vi "Properties Section Page.vi"(8 "error in (no error)":errorcluster, 11 "Node Ptr":T1 format="%.0x") -> (0 "error out":errorcluster)   [LabVIEW 2019, in "SLSC EDS System Explorer.lvlib"]
uses:
  SLSC EDS System Explorer.lvlib
  <vilib>/NI VeriStand/Custom Device API/Custom Device Item Ref.ctl
  Shared/Constants.vi
  <vilib>/NI VeriStand/Custom Device API/Custom Device API.lvlib
  Shared/SLSC EDS Shared.lvlib
panel:
  in  "SHDocVw.IWebBrowser":refnum<k7>(container)
  in  "Header 2":cluster{"Section Name":string}={"Section Name"="Properties Settings"}
  # "Name"
  # "Description"
  # "Datatype"
  # "Value"
  # "Min"
  # "Max"
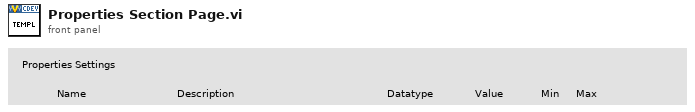
[diagram p1: front panel]
types:
  T1 = typedef "Custom Device API.lvlib/Custom Device Item Ref.ctl" = u64
  T2 = typedef "Custom Device API.lvlib/Custom Device Commands.ctl" = enum16{"Default", "Item renamed", "Shutdown", "Dynamic button pressed"}
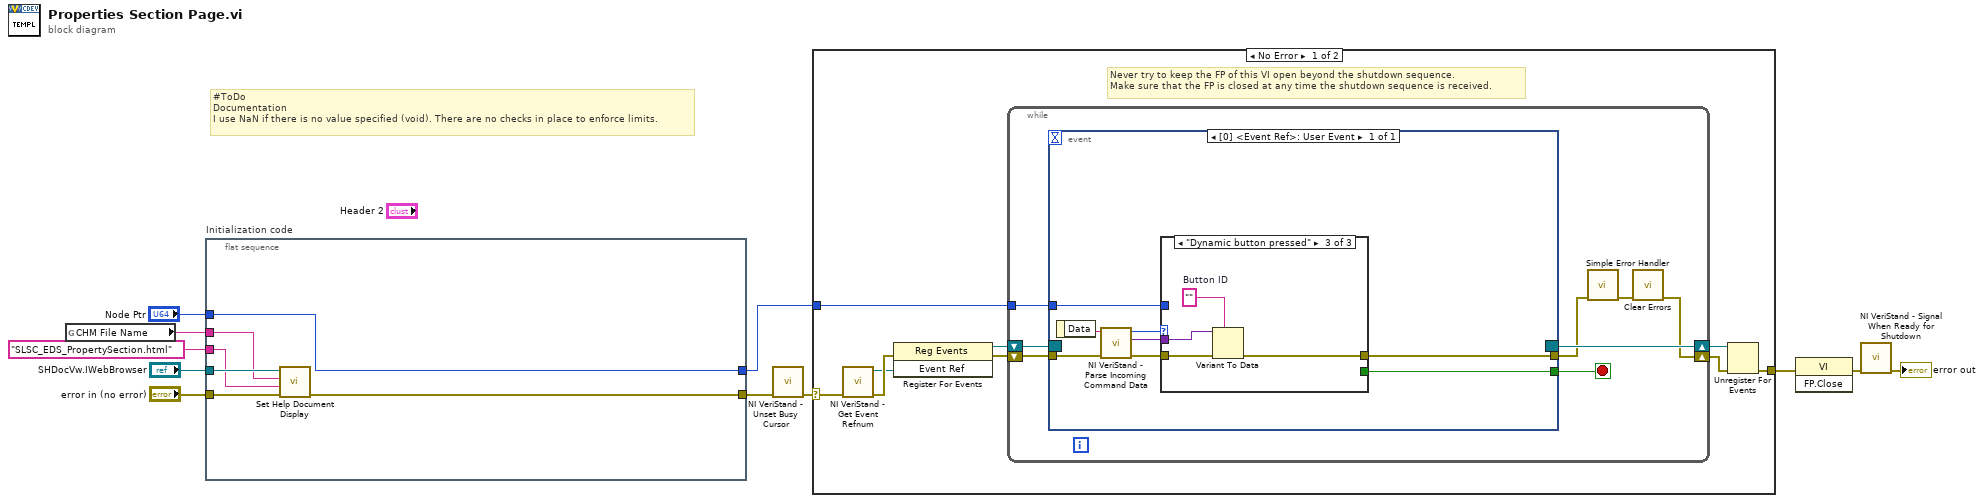
[diagram p0: block diagram]
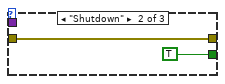
[diagram p3: hidden frame]
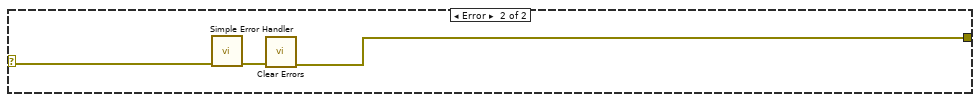
[diagram p4: hidden frame]
diagram:
  # "#ToDo\nDocumentation\nI use NaN if there is no value specified (void). There are no checks in place to enforce limits."
  n1 = global read "Constants.vi" "CHM File Name"() -> (w1:string)
  n2 = flat-sequence "Initialization code" {
    tunnel: "error in (no error)" -> [w17]
    tunnel: "Node Ptr" -> [w13]
    tunnel: [w12] -> w7
    tunnel: [w13] -> w4
    tunnel: "SHDocVw.IWebBrowser" -> [w16]
    tunnel: "SLSC_EDS_PropertySection.html" ("HTML File") -> [w15]
    tunnel: w1 -> [w14]
    frame #0 {
      n3 = call "Set Help Document Display.vi"("error in (no error)"=w17, "HTML File"=w15, "Main CHM File"=w14, "SHDocVw.IWebBrowser2"=w16) -> ("error out"=w12:errorcluster)  [unwired: 7 in]
    }
  }
  n4 = call <vilib>:"NI VeriStand - Unset Busy Cursor.vi"("error in (no error)"=w7) -> ("error out"=w6:errorcluster)  [unwired: 10 out]
  n5 = case shown="No Error" w6 {
    selector: w6 -> [w18 w52]
    tunnel: [w23 w50] -> w11
    tunnel: w4 -> [w19 _]
    frame No Error {
      # "Never try to keep the FP of this VI open beyond the shutdown sequence.\nMake sure that the FP is closed at any time the shutdown sequence is received."
      n6 = call <vilib>:"NI VeriStand - Get Event Refnum.vi"("error in (no error)"=w18) -> ("error out"=w26:errorcluster, "Event Ref"=w22:refnum<user-event>)  [unwired: 9 out]
      n7 = register-events(error in=w26, w22) -> (reference out=w20:refnum<event-registration>, error out=w21:errorcluster)  [unwired: 1 in]
      n8 = while {
        tunnel: w19 -> [w30]
        shift-right: [w27] -> w24
        shift-left: w21 -> [w33]
        shift-right: [w34] -> w25
        shift-left: w20 -> [w32]
        stop <- w31 stop-if-true
        n9 = event shown="[0] <Event Ref>: User Event" {
          selector: w32 -> [_]
          dyn-events: [_] -> w34
          timeout: _ -> [_]
          tunnel: w33 -> [w42]
          tunnel: [w38] -> w31
          tunnel: [w37] -> w29
          tunnel: w30 -> [w36]
          event User Event {
            n10 = event-data() -> ("Data"=w41:string)  [unwired: 1 out]
            n11 = call <vilib>:"NI VeriStand - Parse Incoming Command Data.vi"("error in (no error)"=w42, "Incoming data"=w41) -> ("error out"=w40:errorcluster, "Outgoing data"=w35:variant, "Action"=w39:T2)  [unwired: 7 out]
            n12 = case shown="\"Dynamic button pressed\"" w39 {
              tunnel: w40 -> [w43 w44 w49]
              tunnel: [_ TRUE _] -> w38
              tunnel: [w43 w44 w46] -> w37
              tunnel: w36 -> [_ _ _]
              tunnel: w35 -> [_ _ w48]
              frame "Default", Default {
              }
              frame "Shutdown" {
              }
              frame "Dynamic button pressed" {
                w47 = ""  # Button ID
                n13 = Variant To Data(error in=w49, type=w47, Variant=w48) -> (error out=w46:errorcluster)  [unwired: 1 out]
              }
            }
          }
        }
        n14 = call <vilib>:"Simple Error Handler.vi"("error in (no error)"=w29) -> ("error out"=w28:errorcluster)  [unwired: 1 in, 7 out]
        n15 = call <vilib>:"Clear Errors.vi"("error in (no error)"=w28) -> ("error out"=w27:errorcluster)  [unwired: 1 in, 5 out]
      }
      n16 = Unregister For Events(event registration refnum=w25, error in=w24) -> (error out=w23:errorcluster)
    }
    frame Error {
      n17 = call <vilib>:"Simple Error Handler.vi"("error in (no error)"=w52) -> ("error out"=w51:errorcluster)  [unwired: 1 in, 7 out]
      n18 = call <vilib>:"Clear Errors.vi"("error in (no error)"=w51) -> ("error out"=w50:errorcluster)  [unwired: 1 in, 5 out]
    }
  }
  n19 = invoke class="VI" method="FP.Close"(error in=w11) -> (error out=w10:errorcluster)  [unwired: 2 in, 2 out]
  n20 = call <vilib>:"NI VeriStand - Signal When Ready for Shutdown.vi"("error in (no error)"=w10) -> ("error out"=→"error out":errorcluster)  [unwired: 10 out]
